vi "InitDO.vi"   [LabVIEW 2014]
doc: "this VI should be included in the Begin.vi"
types:
  T1 = typedef "DOs.ctl" = cluster{"DIOChannel":T2, "Name":string}[]
  T2 = typedef "FPGA_DIOChannel.ctl" = enum8{"DIO 1", "DIO 2", "DIO 3", "DIO 4", "DIO 5", "DIO 6", "DIO 7", "DIO 8", "DIO 9", "DIO 10", "DIO 11", "DIO 12", "DIO 13", "DIO 14", "Invalid"}
  T3 = typedef "WPI_DigitalOutputDevRef.ctl" = cluster{"Digital Module":T4, "DIO Channel":T2, "DevStatus":errorcluster}
  T4 = typedef "FPGA_TypedefDigitalModule.ctl" = enum16{"Digital Module 1", "Digital Module 2"}
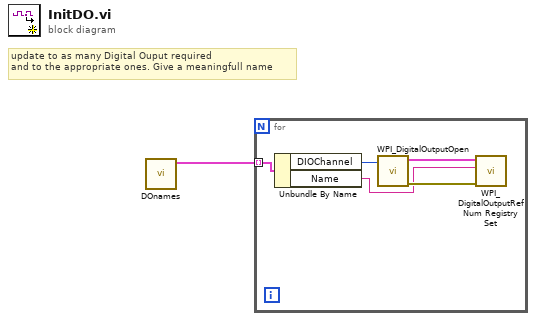
[diagram p0: block diagram]
diagram:
  # "update to as many Digital Ouput required\nand to the appropriate ones. Give a meaningfull name"
  n1 = call "DOnames.vi"() -> ("DIO Channel"=w1:T1)  [unwired: 11 in]
  n2 = for {
    tunnel: w1 -> [w6] mode=indexing
    n3 = Unbundle By Name(w6) -> ("DIOChannel"=w3:T2, "Name"=w2:string)
    n4 = call <vilib>:"WPI_DigitalOutputOpen.vi"("DIO Channel"=w3) -> ("error out"=w5:errorcluster, "DigitalOutputDevRef"=w4:T3)  [unwired: 9 in]
    n5 = call <vilib>:"WPI_DigitalOutputRefNum Registry Set.vi"("error in (no error)"=w5, "refnum name"=w2, "DigitalOutputDevRef"=w4) -> ()  [unwired: 7 in, 2 out]
  }
